vi "PruebaSeq.vi"() -> ()   [LabVIEW 2014, in "MSX-E3711_dll.lvlib"]
uses:
  MSX-E3711_dll.lvlib
  Typedef/Config Data.ctl
  Typedef/Connection Data.ctl
  E:/Repositorio Magnis/INF002/v0/Modules/HAL/Drivers/Sync/ADDI-DATA MSX-E3711/API/MSXE371x.dll
  MSXE371x.dll
  E:/Repositorio Magnis/INF002/v0/Modules/HAL/Drivers/Sync/ADDI-DATA MSX-E3711/API/MXCommon.dll
  MXCommon.dll
panel:
  out "Adq. Sequence.Counter Value":u32[](array[numeric])=[1669, 1669]
  out "Adq. Sequence.Adquisition Value":u32[][](array[numeric])=[[7066158, 5327901, 1163029709], [7066122, 5327839, 1163029709]]
  in  "Transductores":bool[][](array[boolean])=[[TRUE, TRUE]]
  in  "stop":bool
  out "error out":errorcluster
  in  "Connection Data In":T1={"MX371x refnum"=refnum, "IP"="192.168.2.98", "Connection ID "=refnum, "MXCommon refnum"=refnum}
  in  "Error In":errorcluster
  in  "Config Data":T2={"Auto Refresh"={"Average Mode"=0, "Average Value"=0, "Trigger Mask"=0, "Trigger Mode"=0, "Hardware Trigger Edge"=0, "Hardware Trigger Count"=0, "By Trigger Nbr Of Seq To Acquire"=0, "Time stamp"=FALSE, "Analog Output(mm)"=FALSE, "Invert value"=FALSE, "Temperature value"=FALSE, "Incremental counter value"=FALSE, "Diff. mode"=FALSE}, "Gain"=[], "Offset"=[], "Index"=202, "Range"=0.0, "Sequence"={"Nbr Of Sequence"=0, "Nbr Max Sequence To Transfer"=2, "Delay Mode"=0, "Delay Time Unit"=0, "Delay Value"=0, "Trigger Mask"=0, "Trigger Mode"=0, "Hardware Trigger Edge"=0, "Hardware Trigger Count"=0, "By Trigger Nbr Of Seq To Acquire"=0, "Time stamp"=FALSE, "Sequence counter information"=FALSE, "Analog Output(mm)"=FALSE, "Invert value"=FALSE, "Temperature value"=TRUE, "Incremental counter value"=TRUE, "Diff. mode"=FALSE}, "Enable DIO"=FALSE, "IncCounter"={"CounterMode"="1", "CounterOptionDIRECT  "=FALSE, "CounterOptionOthers"=FALSE, "CounterClear "=FALSE}, "IncTemperature"={"ConnectedTempSensor"="100", "ConvertMode"="1", "InitGainSelection"="0", "FrequencySelection"="240", "PowerSaveMode"=FALSE, "GainSelection"="", "RefValue"=0.0}}
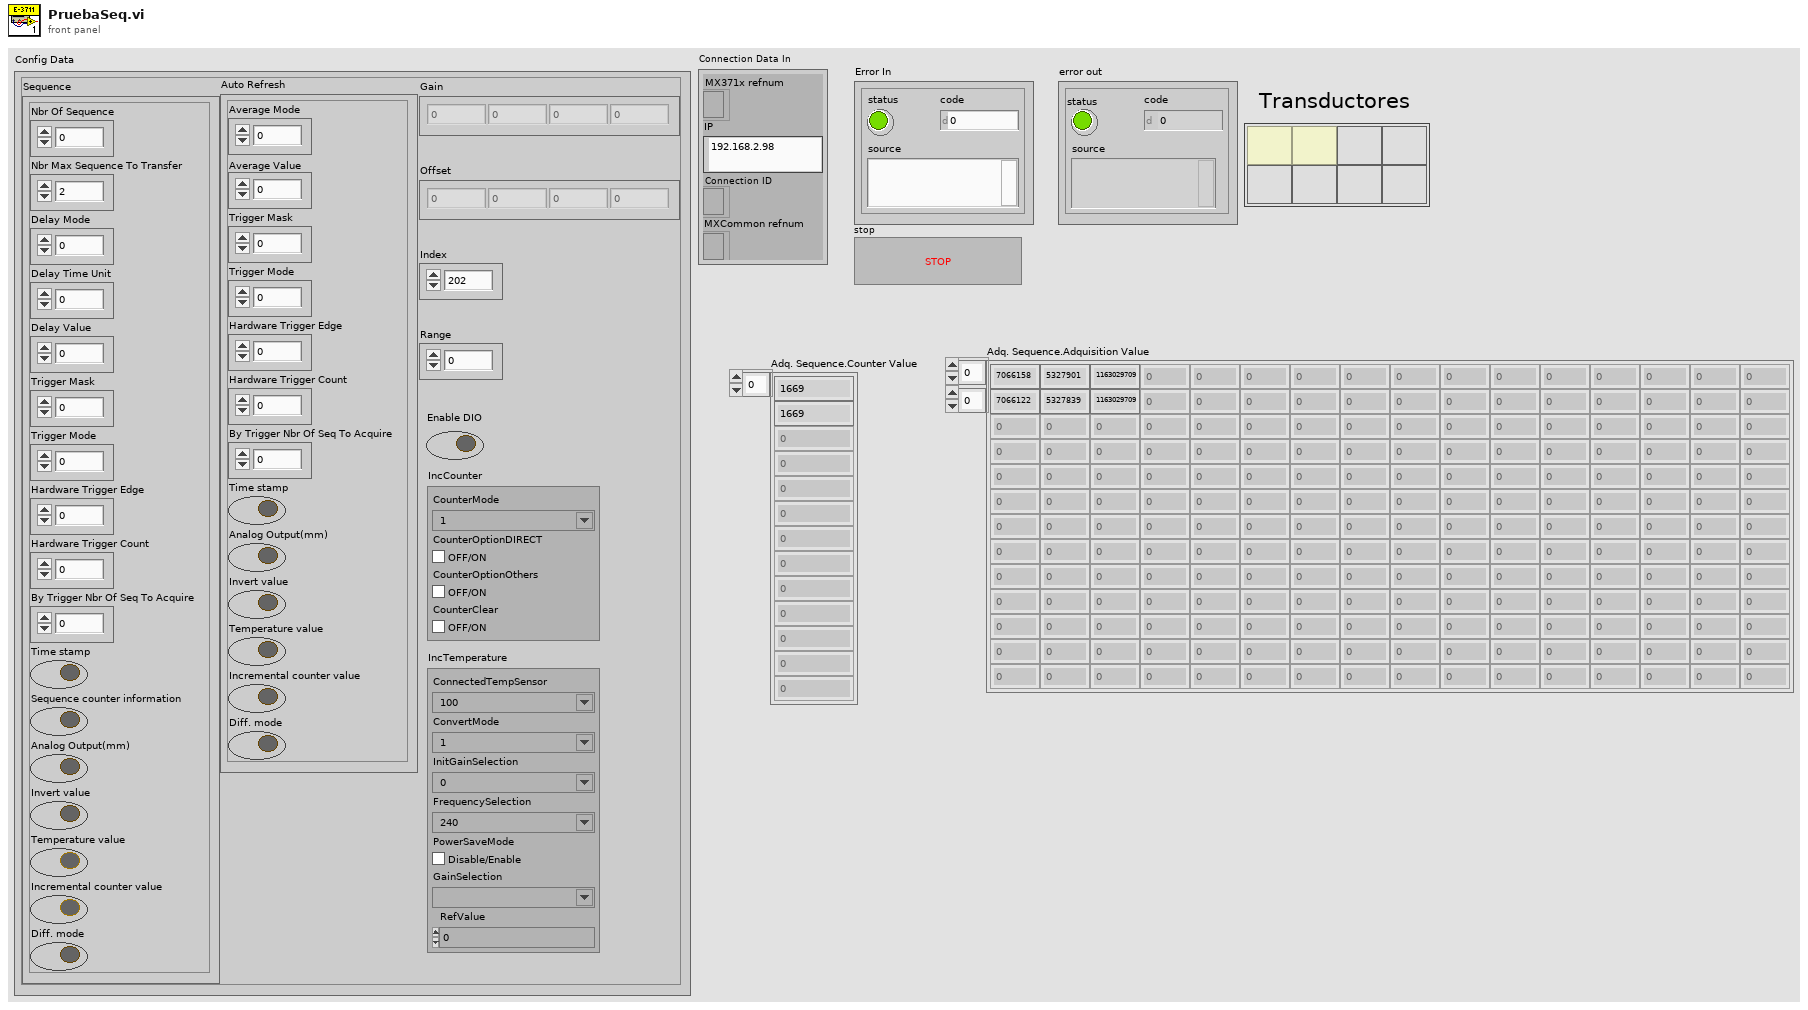
[diagram p1: front panel]
types:
  T1 = typedef "MSX-E3711_dll.lvlib/Connection Data.ctl" = cluster{"MX371x refnum":refnum<k24>, "IP":string, "Connection ID ":refnum<k5>, "MXCommon refnum":refnum<k24>}
  T2 = typedef "MSX-E3711_dll.lvlib/Config Data.ctl" = cluster{"Auto Refresh":cluster{"Average Mode":u64, "Average Value":u64, "Trigger Mask":u64, "Trigger Mode":u64, "Hardware Trigger Edge":u64, "Hardware Trigger Count":u64, "By Trigger Nbr Of Seq To Acquire":u64, "Time stamp":bool, "Analog Output(mm)":bool, "Invert value":bool, "Temperature value":bool, "Incremental counter value":bool, "Diff. mode":bool}, "Gain":sgl[], "Offset":sgl[], "Index":u64, "Range":sgl, "Sequence":cluster{"Nbr Of Sequence":u64, "Nbr Max Sequence To Transfer":u64, "Delay Mode":u64, "Delay Time Unit":u64, "Delay Value":u64, "Trigger Mask":u64, "Trigger Mode":u64, "Hardware Trigger Edge":u64, "Hardware Trigger Count":u64, "By Trigger Nbr Of Seq To Acquire":u64, "Time stamp":bool, "Sequence counter information":bool, "Analog Output(mm)":bool, "Invert value":bool, "Temperature value":bool, "Incremental counter value":bool, "Diff. mode":bool}, "Enable DIO":bool, "IncCounter":cluster{"CounterMode":string, "CounterOptionDIRECT  ":bool, "CounterOptionOthers":bool, "CounterClear ":bool}, "IncTemperature":cluster{"ConnectedTempSensor":string, "ConvertMode":string, "InitGainSelection":string, "FrequencySelection":string, "PowerSaveMode":bool, "GainSelection":string, "RefValue":dbl}}
  T3 = typedef "MSX-E3711_dll.lvlib/Adquisition Data.ctl" = cluster{"Adq. Sequence":cluster{"Adquisition Value":u32[][], "Counter Value":u32[], "TSs - TSu - NAS":u64[][], "Status IO Port":bool[]}, "Adq. Auto Refresh":cluster{"Adquisition Value":u64[], "Status IO Port":bool[], "Counter value":u64}}
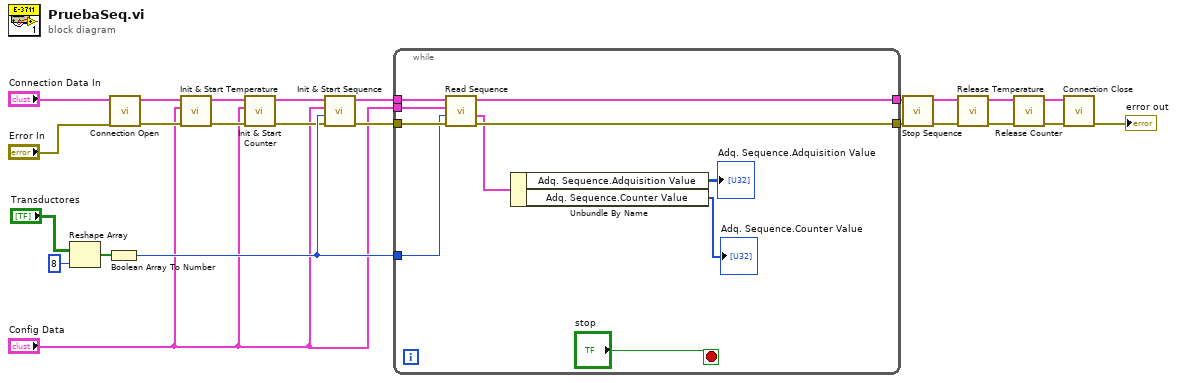
[diagram p0: block diagram]
diagram:
  n1 = Reshape Array("Transductores", 8 ("dimension size")) -> (w17:bool[])
  n2 = Boolean Array To Number(Boolean array=w17) -> (number=w14:u64)
  n3 = call "Connection Open.vi"("error in (no error)"="Error In", "Connection Data In"="Connection Data In") -> ("error out"=w10:errorcluster, "Connection Data Out"=w9:T1)  [unwired: 8 in]
  n4 = call "Init & Start Temperature.vi"("error in (no error)"=w10, "Config Data"="Config Data", "Connection Data In"=w9) -> ("error out"=w11:errorcluster, "Connection Data Out"=w8:T1)  [unwired: 7 in]
  n5 = call "Init & Start Counter.vi"("error in (no error)"=w11, "Config Data"="Config Data", "Connection Data In"=w8) -> ("error out"=w12:errorcluster, "Connection Data Out"=w13:T1)  [unwired: 7 in]
  n6 = call "Init & Start Sequence.vi"("error in (no error)"=w12, "Channel Mask"=w14, "Config Data"="Config Data", "Connection Data In"=w13) -> ("error out"=w19:errorcluster, "Connection Data Out"=w21:T1)  [unwired: 6 in]
  n7 = while {
    tunnel: "Config Data" -> [w30]
    tunnel: w21 -> [w34]
    tunnel: [w33] -> w20
    tunnel: w19 -> [w32]
    tunnel: [w31] -> w18
    tunnel: w14 -> [w28]
    stop <- "stop" stop-if-true
    n8 = call "Read Sequence.vi"("error in (no error)"=w32, "Channel Mask"=w28, "Config Data"=w30, "Connection Data In"=w34) -> ("error out"=w31:errorcluster, "Adquisition Data Out"=w27:T3, "Connection Data Out"=w33:T1)  [unwired: 5 in]
    n9 = Unbundle By Name(w27) -> ("Adq. Sequence.Adquisition Value"=→"Adq. Sequence.Adquisition Value":u32[][], "Adq. Sequence.Counter Value"=→"Adq. Sequence.Counter Value":u32[])
  }
  n10 = call "Stop Sequence.vi"("error in (no error)"=w18, "Connection Data In"=w20) -> ("error out"=w5:errorcluster, "Connection Data Out"=w6:T1)  [unwired: 8 in]
  n11 = call "Release Temperature.vi"("error in (no error)"=w5, "Connection Data In"=w6) -> ("error out"=w3:errorcluster, "Connection Data Out"=w4:T1)  [unwired: 8 in]
  n12 = call "Release Counter.vi"("error in (no error)"=w3, "Connection Data In"=w4) -> ("error out"=w1:errorcluster, "Connection Data Out"=w2:T1)  [unwired: 8 in]
  n13 = call "Connection Close.vi"("error in (no error)"=w1, "Connection Data In"=w2) -> ("error out"=→"error out":errorcluster)  [unwired: 8 in, 1 out]
